vi "IBM4_Diff_Read(V1).vi"(8 "error in":errorcluster, 9 "Neg-Chan":i32=1, 10 "Pos-Chan":i32, 11 "COM resource in":refnum<visa-resource-name>="COM9") -> (0 "error out":errorcluster, 2 "output":dbl, 3 "COM resource out":refnum<visa-resource-name>)   [LabVIEW 2021, in "IBM4.lvlib"]
doc: "This VI interfaces with the IBM4 to perform a differential read operation.\n\nThe input channels must be between 0 and 4, while the output will be in floating point format (thus, in Volts).\nOnly a single read operation is made with this VI. \n\nAlternate read operations exist covering binary or floating point, single reading, multiple readings, and an average of multiple readings (floating point only)."
uses:
  <instrlib>/IBM4/IBM4.lvlib
panel:
  out "error out 2":errorcluster
  out "read buffer":string
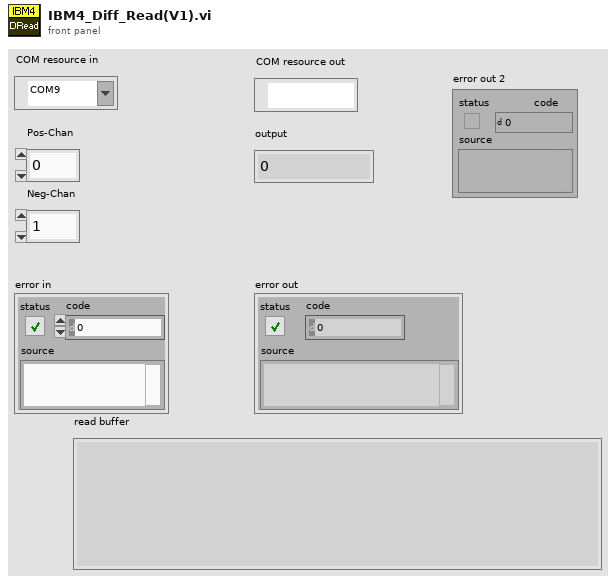
[diagram p1: front panel]
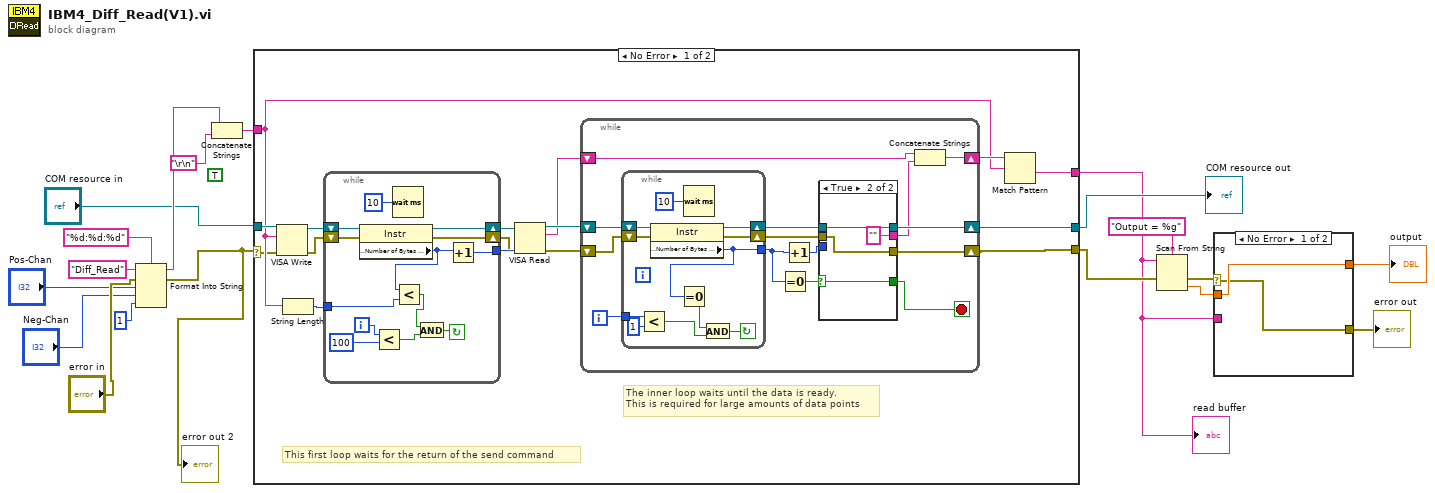
[diagram p0: block diagram]
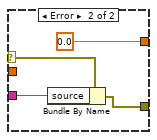
[diagram p2: hidden frame]
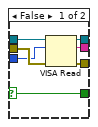
[diagram p3: hidden frame]
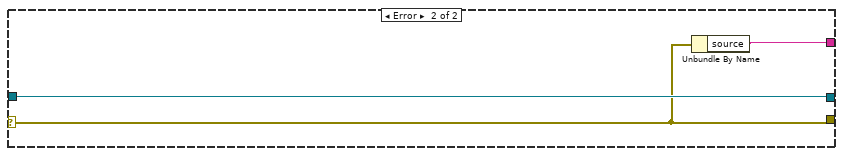
[diagram p4: hidden frame]
diagram:
  (unwired) TRUE ("Enable Termination\nChar (T)")
  n1 = Format Into String(format string="%d:%d:%d", initial string="Diff_Read", error in="error in", "Pos-Chan", "Neg-Chan", 1 ("input 2")) -> (resulting string=w11:string, error out=w1:errorcluster)
  "error out 2" <- w1
  n2 = Concatenate Strings(w11, "\r\n") -> (w10:string)
  n3 = case shown="No Error" w1 {
    selector: w1 -> [w22 w85]
    tunnel: "COM resource in" -> [w35 w87]
    tunnel: [w21 w85] -> w14
    tunnel: [w33 w86] -> w6
    tunnel: w10 -> [w32 _]
    tunnel: [w20 w87] -> w15
    frame No Error {
      # "The inner loop waits until the data is ready.\nThis is required for large amounts of data points"
      # "This first loop waits for the return of the send command"
      n4 = VISA Write(VISA resource name=w35, write buffer=w32, error in (no error)=w22) -> (VISA resource name out=w31:refnum<visa-resource-name>, error out=w30:errorcluster)  [unwired: 1 out]
      n5 = String Length(string=w32) -> (length=w23:i32)
      n6 = while {
        tunnel: [w37] -> w28
        shift-right: [w47] -> w29
        shift-left: w31 -> [w48]
        shift-right: [w45] -> w27
        shift-left: w30 -> [w46]
        tunnel: w23 -> [w43]
        i -> [w38]
        stop <- w41 continue-if-true
        n7 = property class="Instr"(reference=w48, error in=w46) -> (reference out=w47:refnum<visa-resource-name>, error out=w45:errorcluster, "Serial Settings:Number of Bytes at Serial Port"=w36:u32)
        n8 = Less?(x=w38, y=100) -> (x < y?=w40:bool)
        n9 = Wait (ms)(milliseconds to wait=u32 10) -> ()  [unwired: 1 out]
        n10 = Less?(x=w36, y=w43) -> (x < y?=w39:bool)
        n11 = And(x=w39, y=w40) -> (x .and. y?=w41:bool)
        n12 = Increment(x=w36) -> (x+1=w37:u32)
      }
      n13 = VISA Read(VISA resource name=w29, byte count=w28, error in (no error)=w27) -> (VISA resource name out=w26:refnum<visa-resource-name>, read buffer=w24:string, error out=w25:errorcluster)  [unwired: 1 out]
      n14 = while {
        shift-right: [w62] -> w20
        shift-left: w26 -> [w60]
        shift-right: [w61] -> w21
        shift-left: w25 -> [w58]
        shift-right: [w56] -> w34
        shift-left: w24 -> [w54]
        i -> [w53]
        stop <- w49 stop-if-true
        n15 = while {
          tunnel: [w79] -> w52
          shift-right: [w83] -> w59
          shift-left: w60 -> [w84]
          shift-right: [w81] -> w57
          shift-left: w58 -> [w82]
          tunnel: w53 -> [w78]
          stop <- w76 continue-if-true
          n16 = Less?(x=w78, y=1) -> (x < y?=w75:bool)
          n17 = property class="Instr"(reference=w84, error in=w82) -> (reference out=w83:refnum<visa-resource-name>, error out=w81:errorcluster, "Serial Settings:Number of Bytes at Serial Port"=w79:u32)
          n18 = Equal To 0?(x=w79) -> (x = 0?=w74:bool)
          n19 = Wait (ms)(milliseconds to wait=u32 10) -> ()  [unwired: 1 out]
          n20 = And(x=w74, y=w75) -> (x .and. y?=w76:bool)
        }
        n21 = Equal To 0?(x=w52) -> (x = 0?=w50:bool)
        n22 = Increment(x=w52) -> (x+1=w51:u32)
        n23 = case shown="True" w50 {
          selector: w50 -> [w63 w72]
          tunnel: [w69 w73] -> w62
          tunnel: [w68 w71] -> w61
          tunnel: w59 -> [w67 w73]
          tunnel: w57 -> [w66 w71]
          tunnel: [w65 "" ("read buffer")] -> w55
          tunnel: w51 -> [w64 _]
          tunnel: [w63 w72] -> w49
          frame False {
            n24 = VISA Read(VISA resource name=w67, byte count=w64, error in (no error)=w66) -> (VISA resource name out=w69:refnum<visa-resource-name>, read buffer=w65:string, error out=w68:errorcluster)  [unwired: 1 out]
          }
          frame True {
          }
        }
        n25 = Concatenate Strings(w54, w55) -> (w56:string)
      }
      n26 = Match Pattern(string=w34, regular expression=w32) -> (after substring=w33:string)  [unwired: 1 in, 3 out]
    }
    frame Error {
      n27 = Unbundle By Name(w85) -> ("source"=w86:string)
    }
  }
  "COM resource out" <- w15
  "read buffer" <- w6
  n28 = Scan From String(format string="Output = %g", input string=w6, error in=w14) -> (error out=w9:errorcluster, output 1=w3:dbl)  [unwired: 2 in, 2 out]
  n29 = case shown="No Error" w9 {
    selector: w9 -> [w88 w92]
    tunnel: w3 -> [w89 _]
    tunnel: [w89 0.0] -> w8
    tunnel: [w88 w90] -> w7
    tunnel: w6 -> [_ w91]
    frame No Error {
    }
    frame Error {
      n30 = Bundle By Name(cluster=w92, "source"=w91) -> (w90:errorcluster)
    }
  }
  "error out" <- w7
  "output" <- w8
